vi "Time_FGV_test.vi"() -> ()   [LabVIEW 2017]
panel:
  out "경과시간 2":dbl
  out "경과시간":dbl
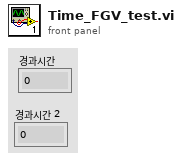
[diagram p1: front panel]
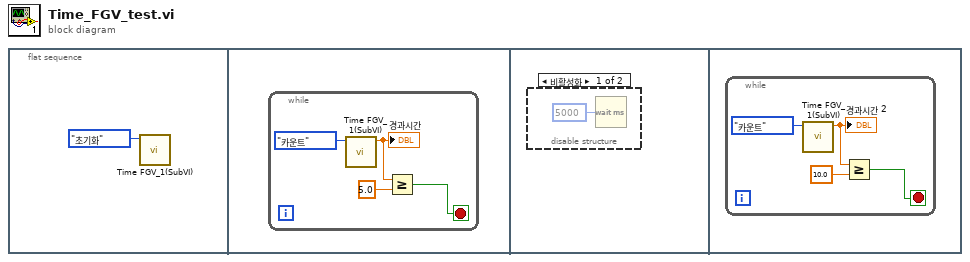
[diagram p0: block diagram]
diagram:
  n1 = flat-sequence {
    frame #0 {
      n2 = call "Time FGV_1(SubVI).vi"("상태"=enum16{"초기화", "카운트", "정지"}."초기화" ("열거형")) -> ()  [unwired: 10 in, 1 out]
    }
    frame #1 {
      n3 = while {
        stop <- w2 stop-if-true
        n4 = call "Time FGV_1(SubVI).vi"("상태"=enum16{"초기화", "카운트", "정지"}."카운트" ("열거형")) -> ("경과시간"=w4:dbl)  [unwired: 10 in]
        "경과시간" <- w4
        n5 = Greater Or Equal?(x=w4, y=5.0) -> (x >= y?=w2:bool)
      }
    }
    frame #2 {
      n6 = disable-structure shown="비활성화" {
        frame Disabled {
          n7 = Wait (ms)(milliseconds to wait=u32 5000 ("대기 시간 (ms)")) -> ()  [unwired: 1 out]
        }
        frame Enabled {
        }
      }
    }
    frame #3 {
      n8 = while {
        stop <- w7 stop-if-true
        n9 = call "Time FGV_1(SubVI).vi"("상태"=enum16{"초기화", "카운트", "정지"}."카운트" ("열거형")) -> ("경과시간"=w9:dbl)  [unwired: 10 in]
        "경과시간 2" <- w9
        n10 = Greater Or Equal?(x=w9, y=10.0) -> (x >= y?=w7:bool)
      }
    }
  }
